vi "Create_Object.vi"(8 "error in (no error)":errorcluster, 9 "Block Diagram in":T1, 10 "owner refnum":variant, 11 "While Loop in":refnum<class "While Loop.lvclass">) -> (0 "error out":errorcluster, 1 "Block Diagram Out":T1, 3 "While Loop out":refnum<class "While Loop.lvclass">)   [LabVIEW 2025, in "While Loop.lvclass"]
uses:
  While Loop.lvclass
  C:/Users/mrjak/Documents/GitHub/LVGPT/LabVIEW/VIs/Classes/Node/Node.lvclass
  Controls/bd.ctl
  Node.lvclass
  Controls/wire.ctl
  Controls/Terminal.ctl
  Node.lvclass/Node.ctl
  Loop.lvclass
  While Loop.lvclass/While Loop.ctl
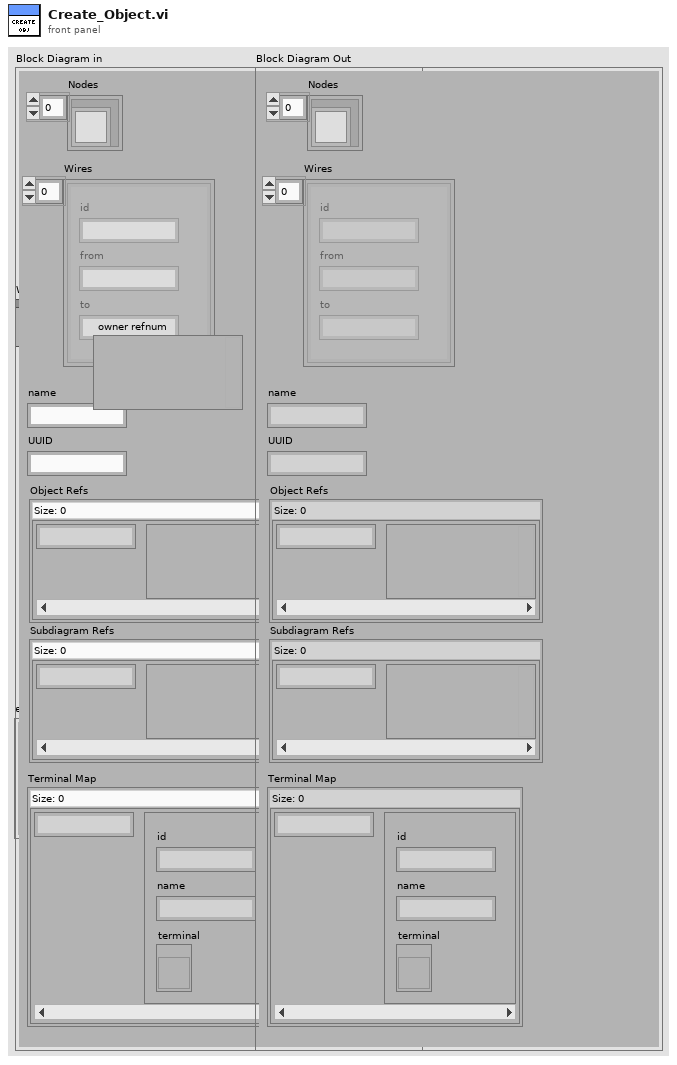
[diagram p1: front panel]
types:
  T1 = typedef "bd.ctl" = cluster{"Nodes":refnum<class "Node.lvclass">[], "Wires":T2[], "name":string, "UUID":string, "Object Refs":map{string, variant}, "Subdiagram Refs":map{string, variant}, "Terminal Map":map{string, T3}}
  T2 = typedef "wire.ctl" = cluster{"id":string, "from":string, "to":string}
  T3 = typedef "Terminal.ctl" = cluster{"id":string, "name":string, "terminal":refnum<vi>}
  T4 = typedef "Subdiagram.ctl" = cluster{"diagram":refnum<vi>, "selector":string, "uuid":string}
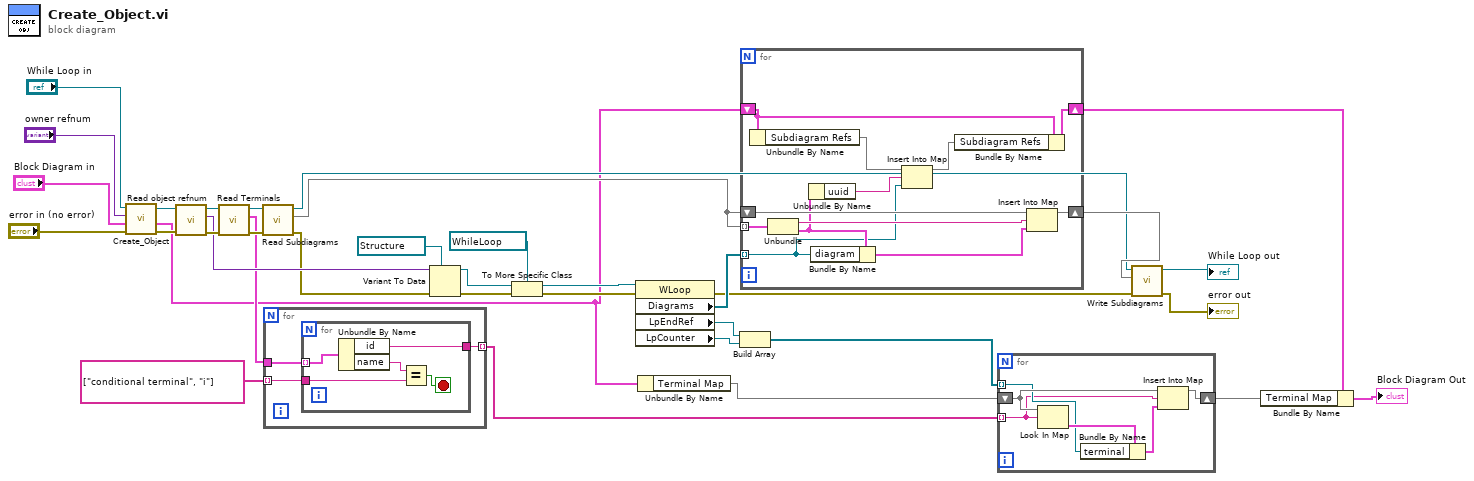
[diagram p0: block diagram]
diagram:
  n1 = call-parent "Create_Object.vi"("error in (no error)"="error in (no error)", "Block Diagram in"="Block Diagram in", "owner refnum"="owner refnum", "Loop in"="While Loop in") -> ("error out"=w15:errorcluster, "Block Diagram Out"=w2:T1, "Loop out"=w14:refnum<class "While Loop.lvclass">)  [unwired: 5 in]
  n2 = call-dynamic "Read object refnum.vi"("error in (no error)"=w15, "Node in"=w14) -> ("error out"=w31:errorcluster, "object refnum"=w21:variant, "Node out"=w32:refnum<class "While Loop.lvclass">)  [unwired: 7 in]
  n3 = call "Read Terminals.vi"("error in (no error)"=w31, "Node in"=w32) -> ("error out"=w22:errorcluster, "Terminals"=w11:T3[], "Node out"=w27:refnum<class "While Loop.lvclass">)  [unwired: 7 in]
  n4 = call-dynamic "Read Subdiagrams.vi"("error in (no error)"=w22, "Structure in"=w27) -> ("error out"=w20:errorcluster, "Subdiagrams"=w26:map{string, T4}, "Structure out"=w24:refnum<class "While Loop.lvclass">)  [unwired: 7 in]
  n5 = for {
    tunnel: w11 -> [w39]
    tunnel: [w38] -> w10 mode=indexing
    tunnel: string[] ["conditional terminal", "i"] -> [w37] mode=indexing
    n6 = for {
      tunnel: w39 -> [w44] mode=indexing
      tunnel: [w42] -> w38
      tunnel: w37 -> [w41]
      stop <- w40 stop-if-true
      n7 = Unbundle By Name(w44) -> ("id"=w42:string, "name"=w43:string)
      n8 = Equal?(x=w43, y=w41) -> (x = y?=w40:bool)
    }
  }
  n9 = Variant To Data(error in=w20, type=refnum<vi> refnum ("vi object class"), Variant=w21) -> (data=w16:refnum<vi>, error out=w19:errorcluster)
  n10 = To More Specific Class(target class=refnum<vi> refnum ("vi object class"), reference=w16, error in=w19) -> (specific class reference=w30:refnum<vi>, error out=w25:errorcluster)
  n11 = property class="WLoop"(reference=w30, error in=w25) -> (error out=w23:errorcluster, "Diagrams"=w29:refnum<vi>[], "LpEndRef"=w8:refnum<vi>, "LpCounter"=w7:refnum<vi>)  [unwired: 1 out]
  n12 = Unbundle By Name(w2) -> ("Terminal Map"=w5:map{string, T3})
  n13 = Build Array(w8, w7) -> (w6:refnum<vi>[])
  n14 = for {
    tunnel: w29 -> [w45] mode=indexing
    tunnel: w26 -> [w56] mode=indexing
    shift-right: [w52] -> w28
    shift-left: w26 -> [w55]
    shift-right: [w50] -> w1
    shift-left: w2 -> [w51]
    n15 = Unbundle By Name(w51) -> ("Subdiagram Refs"=w49:map{string, variant})
    n16 = Unbundle(w56) -> ("String"=w53:string, "Subdiagram"=w47:T4)
    n17 = Unbundle By Name(w47) -> ("uuid"=w46:string)
    n18 = Bundle By Name(cluster=w47, "diagram"=w45) -> (w54:T4)
    n19 = Insert Into Map(map in=w49, key=w46, value=w45) -> (map out=w48:map{string, variant})  [unwired: 2 out]
    n20 = Bundle By Name(cluster=w51, "Subdiagram Refs"=w48) -> (w50:T1)
    n21 = Insert Into Map(map in=w55, key=w53, value=w54) -> (map out=w52:map{string, T4})  [unwired: 2 out]
  }
  n22 = for {
    tunnel: w6 -> [w60] mode=indexing
    tunnel: w10 -> [w57] mode=indexing
    shift-right: [w58] -> w4
    shift-left: w5 -> [w62]
    n23 = Look In Map(map=w62, key=w57) -> (value=w61:T3)  [unwired: 1 in, 1 out]
    n24 = Bundle By Name(cluster=w61, "terminal"=w60) -> (w59:T3)
    n25 = Insert Into Map(map in=w62, key=w57, value=w59) -> (map out=w58:map{string, T3})  [unwired: 2 out]
  }
  n26 = call-dynamic "Write Subdiagrams.vi"("error in (no error)"=w23, "Subdiagrams"=w28, "Structure in"=w24) -> ("error out"=→"error out":errorcluster, "Structure out"=→"While Loop out":refnum<class "While Loop.lvclass">)  [unwired: 7 in]
  n27 = Bundle By Name(cluster=w1, "Terminal Map"=w4) -> (→"Block Diagram Out":T1)
